vi "Adjust Baselines For Selected Record.vi"(1 "Extension Baseline (nm)":dbl, 2 "Force Baseline (pN)":dbl, 3 "Input State":T1=[{"Base Directory"=path "", "Experimental Data"={"Experimental Data"={"Extension (nm)"=[], "Force (pN)"=[], "Name"=""}, "Enabled"=FALSE}, "Chain Fit"={"Experimental Data"={"Extension (nm)"=[], "Force (pN)"=[], "Name"=""}, "Enabled"=FALSE}, "Selected"=FALSE, "Ramp Rate (nm/s)"=0.0, "Spring Constant (pN/nm)"=0.0, "Slope (nm/V)"=0.0}]) -> (0 "Adjusted State":T1)   [LabVIEW 2013]
uses:
  Analysis Data.ctl
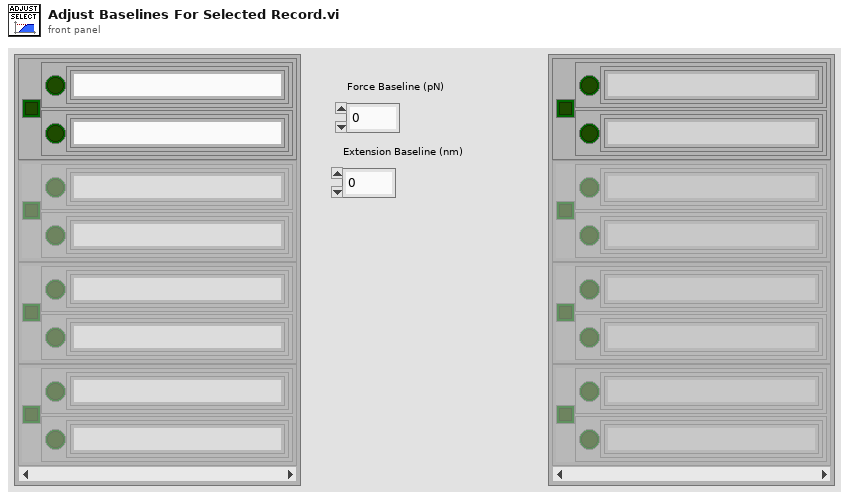
[diagram p1: front panel]
types:
  T1 = typedef "Analysis Data.ctl" = cluster{"Base Directory":path, "Experimental Data":cluster{"Experimental Data":cluster{"Extension (nm)":dbl[], "Force (pN)":dbl[], "Name":string}, "Enabled":bool}, "Chain Fit":cluster{"Experimental Data":cluster{"Extension (nm)":dbl[], "Force (pN)":dbl[], "Name":string}, "Enabled":bool}, "Selected":bool, "Ramp Rate (nm/s)":dbl, "Spring Constant (pN/nm)":dbl, "Slope (nm/V)":dbl}[]
  T2 = cluster{"Experimental Data":cluster{"Extension (nm)":dbl[], "Force (pN)":dbl[], "Name":string}, "Enabled":bool}
  T3 = cluster{"Base Directory":path, "Experimental Data":cluster{"Experimental Data":cluster{"Extension (nm)":dbl[], "Force (pN)":dbl[], "Name":string}, "Enabled":bool}, "Chain Fit":cluster{"Experimental Data":cluster{"Extension (nm)":dbl[], "Force (pN)":dbl[], "Name":string}, "Enabled":bool}, "Selected":bool, "Ramp Rate (nm/s)":dbl, "Spring Constant (pN/nm)":dbl, "Slope (nm/V)":dbl}
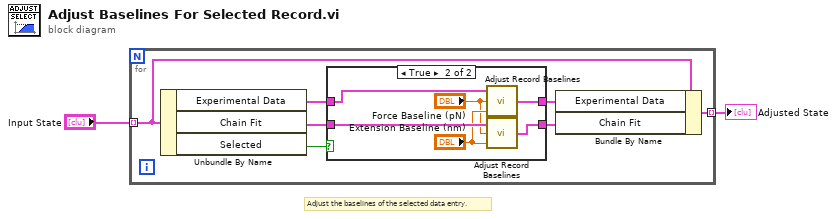
[diagram p0: block diagram]
diagram:
  # "Adjust the baselines of the selected data entry."
  n1 = for {
    tunnel: "Input State" -> [w6] mode=indexing
    tunnel: [w3] -> w1 mode=indexing
    n2 = Unbundle By Name(w6) -> ("Experimental Data"=w9:T2, "Chain Fit"=w8:T2, "Selected"=w7:bool)
    n3 = case shown="True" w7 {
      tunnel: w8 -> [w10 w16]
      tunnel: w9 -> [w11 w17]
      tunnel: [w10 w12] -> w4
      tunnel: [w11 w13] -> w5
      frame False {
      }
      frame True {
        n4 = call "Adjust Record Baselines.vi"("Extension Baseline (nm)"="Extension Baseline (nm)", "Force Baseline (pN)"="Force Baseline (pN)", "Record"=w17) -> ("Adjusted Record"=w13:T2)
        n5 = call "Adjust Record Baselines.vi"("Extension Baseline (nm)"="Extension Baseline (nm)", "Force Baseline (pN)"="Force Baseline (pN)", "Record"=w16) -> ("Adjusted Record"=w12:T2)
      }
    }
    n6 = Bundle By Name(cluster=w6, "Experimental Data"=w5, "Chain Fit"=w4) -> (w3:T3)
  }
  "Adjusted State" <- w1
